vi "Test Comm Multi.vi"() -> ()   [LabVIEW 2021]
uses:
  ChannelCommon/typedef/FIFO Config.ctl
  ChannelCommon/ChannelCommon.lvlib
  CIFChannels/Typedef/Direction.ctl
  CIFChannels/CIFChannels.lvclass
  ChannelCommon/typedef/TimeStamps.ctl
  CIF_Fifo_U8_Multi.lvclass
  ChannelCommon/typedef/New FIFO Instance Configuration.ctl
  FIFO_U8/CIF_NIChn_Fifo_U8.lvclass
  D:/dev/Packages/CIF_Channels_Core/src/CIF_NIChn/FIFO_U8/CIF_NIChn_Fifo_U8.lvclass
  D:/dev/Packages/CIF_Channels_Core/src/CIF_NIChn/NIChn/CIF_NIChn.lvclass
  D:/dev/Packages/CIF_Channels_Core/src/CIFChannels/CIFChannels.lvclass
  D:/dev/Packages/CIF_Channels_Core/src/CIF_NIChn/FIFO_U8_Multi/CIF_Fifo_U8_Multi.lvclass
panel:
  out "status":string
  out "pass":bool
  out "error out":errorcluster
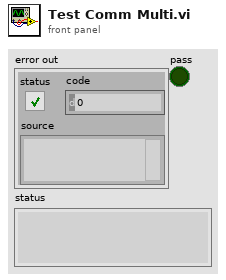
[diagram p1: front panel]
types:
  T1 = typedef "CIFChannels.lvclass/Direction.ctl" = enum16{"Publisher", "Subscriber"}
  T2 = typedef "ChannelCommon.lvlib/New FIFO Instance Configuration.ctl" = cluster{"Primary":bool, "Backpressure":bool, "Message/FIFO Override":u32}
  T3 = typedef "ChannelCommon.lvlib/TimeStamps.ctl" = cluster{"ClockID":u8, "T0":i64, "T_Out":i64}
  T4 = typedef "ChannelCommon.lvlib/FIFO Config.ctl" = cluster{"Max Bytes/Msg":u64, "Max Msg/FIFO":u64, "Flags":u64}
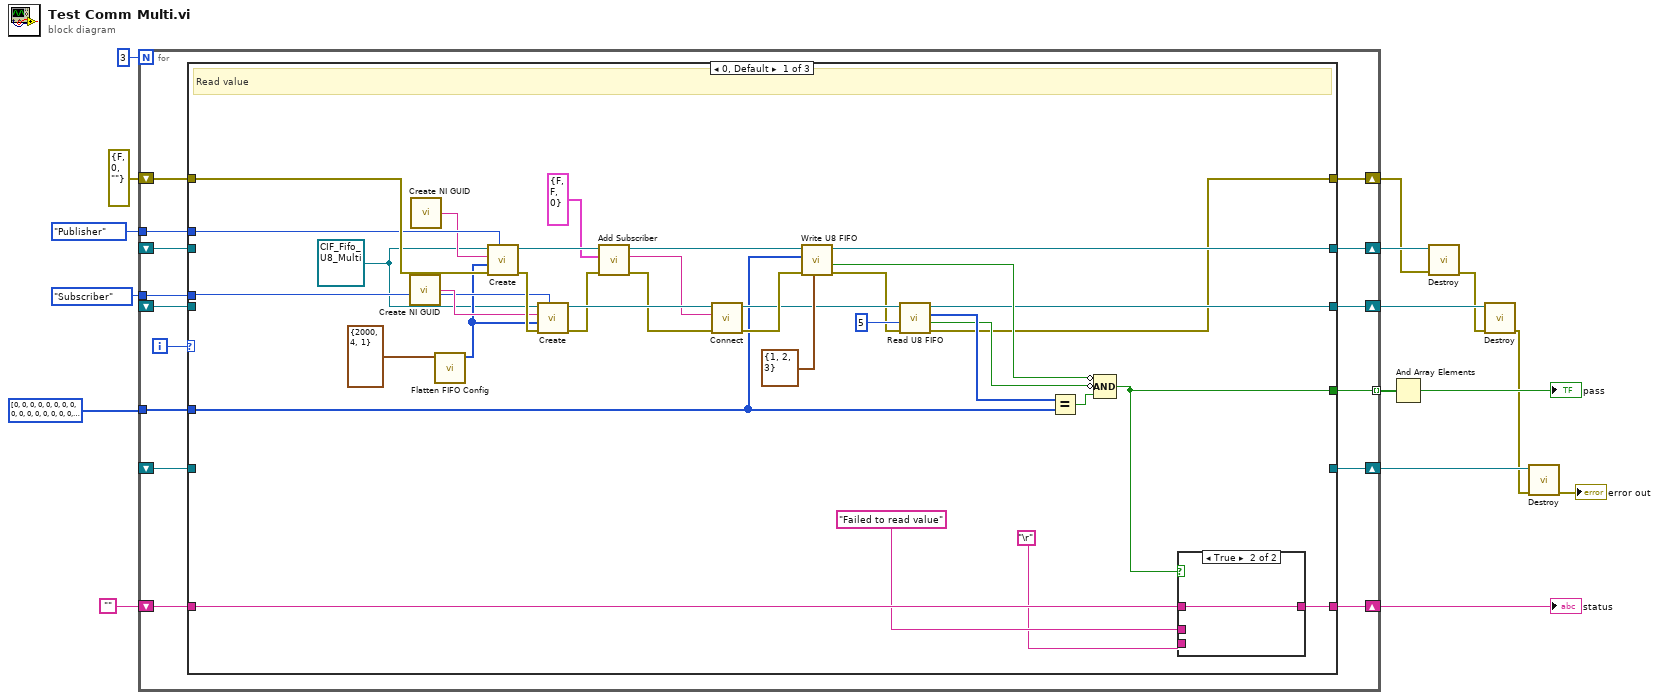
[diagram p0: block diagram]
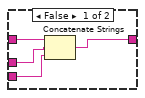
[diagram p2: hidden frame]
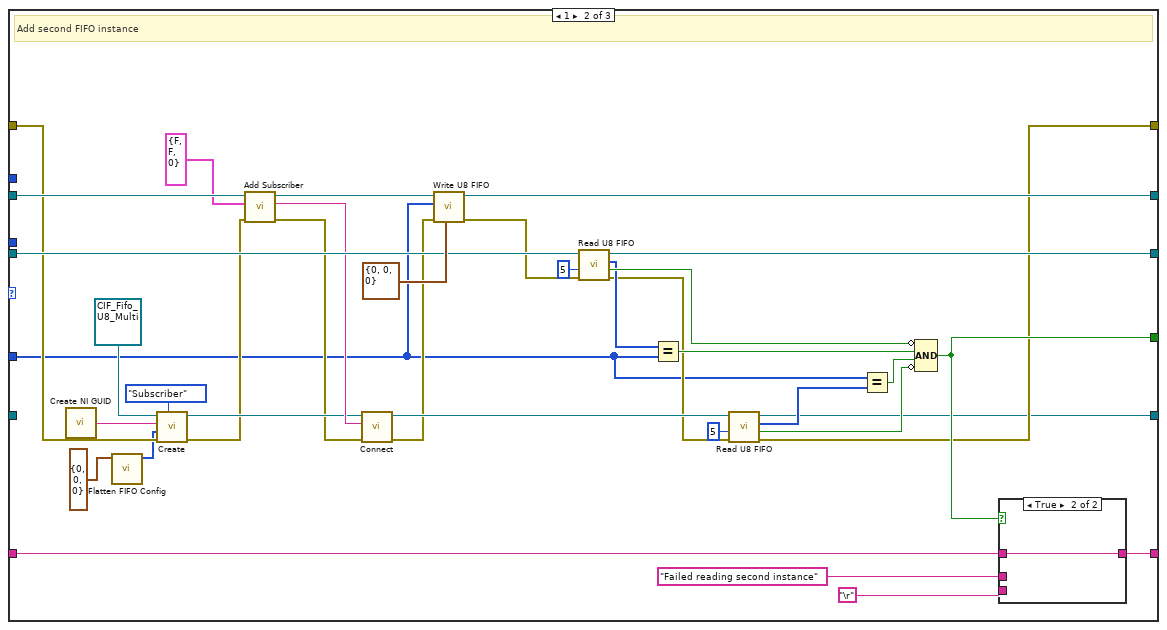
[diagram p3: hidden frame]
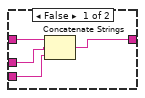
[diagram p4: hidden frame]
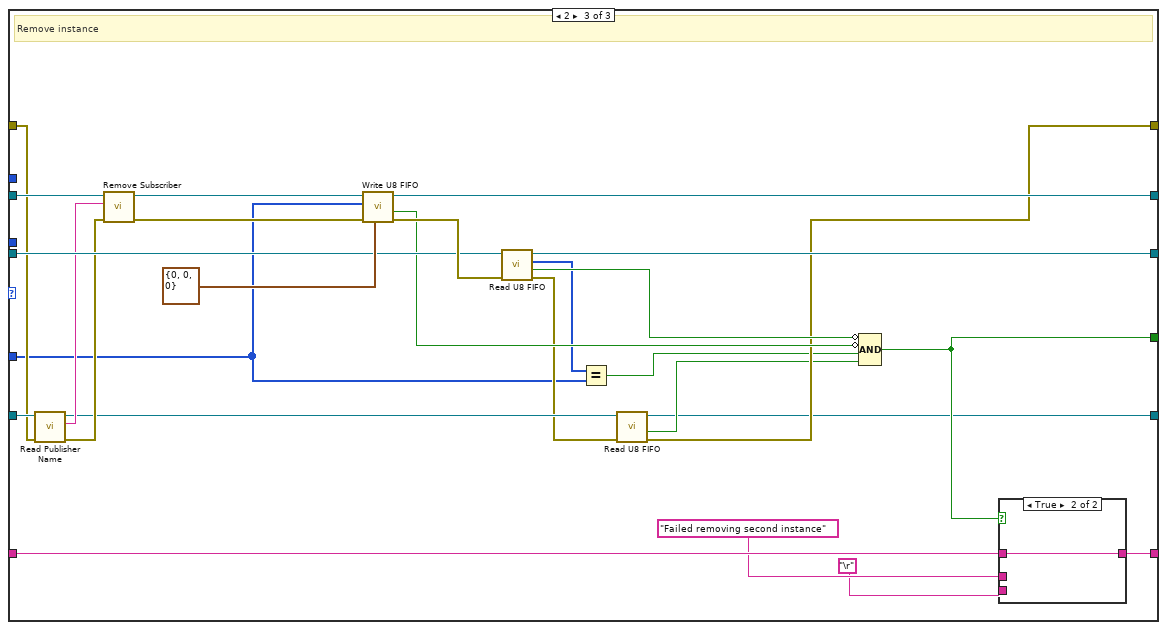
[diagram p5: hidden frame]
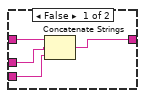
[diagram p6: hidden frame]
diagram:
  n1 = for {
    N: 3 -> [_]
    tunnel: [w31] -> w16 mode=indexing
    shift-right: [w22] -> w6
    shift-left: errorcluster {"status"=FALSE, "code"=0, "source"=""} ("error out") -> [w30]
    shift-right: [w27] -> w12
    shift-left: "" -> [w28]
    tunnel: Direction."Subscriber" ("Direction") -> [w26]
    tunnel: Direction."Publisher" ("Direction") -> [w25]
    shift-right: [w24] -> w8
    shift-left: _ -> [w20]
    shift-right: [w23] -> w7
    shift-left: _ -> [w21]
    tunnel: u8[] [0, 0, 0, 0, 0, 0, 0, 0, 0, 0, 0, 0, 0, 0, 0, 0, 0, 0, 0, 0, 0, 0, 0, 0, 0, 0, 0, 0, 0, 0, 0, 0, 0, 0, 0, 0, 0, 0, 0, 0, 0, 0, 0, 0, 0, 0, 0, 0, 0, 0, 0, 0, 0, 0, 0, 0, 0, 0, 0, 0, 0, 0, 0, 0, 0, 0, 0, 0, 0, 0, 0, 0, 0, 0, 0, 0, 0, 0, 0, 0, 0, 0, 0, 0, 0, 0, 0, 0, 0, 0, 0, 0, 0, 0, 0, 0, 0, 0, 0, 0, 0, 0, 0, 0, 0, 0, 0, 0, 0, 0, 0, 0, 0, 0, 0, 0, 0, 0, 0, 0, 0, 0, 0, 0, 0, 0, 0, 0, 0, 0, 0, 0, 0, 0, 0, 0, 0, 0, 0, 0, 0, 0, 0, 0, 0, 0, 0, 0, 0, 0, 0, 0, 0, 0, 0, 0, 0, 0, 0, 0, 0, 0, 0, 0, 0, 0, 0, 0, 0, 0, 0, 0, 0, 0, 0, 0, 0, 0, 0, 0, 0, 0, 0, 0, 0, 0, 0, 0, 0, 0, 0, 0, 0, 0, 0, 0, 0, 0, 0, 0, 0, 0, 0, 0, 0, 0, 0, 0, 0, 0, 0, 0, 0, 0, 0, 0, 0, 0, 0, 0, 0, 0, 0, 0, 0, 0, 0, 0, 0, 0, 0, 0, 0, 0, 0, 0, 0, 0, 0, 0, 0, 0, 0, 0, 0, 0, 0, 0, 0, 0, 0, 0, 0, 0, 0, 0, 0, 0, 0, 0, 0, 0, 0, 0, 0, 0, 0, 0, 0, 0, 0, 0, 0, 0, 0, 0, 0, 0, 0, 0, 0, 0, 0, 0, 0, 0, 0, 0, 0, 0, 0, 0, 0, 0, 0, 0, 0, 0, 0, 0, 0, 0, 0, 0, 0, 0, 0, 0, 0, 0, 0, 0, 0, 0, 0, 0, 0, 0, 0, 0, 0, 0, 0, 0, 0, 0, 0, 0, 0, 0, 0, 0, 0, 0, 0, 0, 0, 0, 0, 0, 0, 0, 0, 0, 0, 0, 0, 0, 0, 0, 0, 0, 0, 0, 0, 0, 0, 0, 0, 0, 0, 0, 0, 0, 0, 0, 0, 0, 0, 0, 0, 0, 0, 0, 0, 0, 0, 0, 0, 0, 0, 0, 0, 0, 0, 0, 0, 0, 0, 0, 0, 0, 0, 0, 0, 0, 0, 0, 0, 0, 0, 0, 0, 0, 0, 0, 0, 0, 0, 0, 0, 0, 0, 0, 0, 0, 0, 0, 0, 0, 0, 0, 0, 0, 0, 0, 0, 0, 0, 0, 0, 0, 0, 0, 0, 0, 0, 0, 0, 0, 0, 0, 0, 0, 0, 0, 0, 0, 0, 0, 0, 0, 0, 0, 0, 0, 0, 0, 0, 0, 0, 0, 0, 0, 0, 0, 0, 0, 0, 0, 0, 0, 0, 0, 0, 0, 0, 0, 0, 0, 0, 0, 0, 0, 0, 0, 0, 0, 0, 0, 0, 0, 0, 0, 0, 0, 0, 0, 0, 0, 0, 0, 0, 0, 0, 0, 0, 0, 0, 0, 0, 0, 0, 0, 0, 0, 0, 0, 0, 0, 0, 0, 0, 0, 0, 0, 0, 0, 0, 0, 0, 0, 0, 0, 0, 0, 0, 0, 0, 0, 0, 0, 0, 0, 0, 0, 0, 0, 0, 0, 0, 0, 0, 0, 0, 0, 0, 0, 0, 0, 0, 0, 0, 0, 0, 0, 0, 0, 0, 0, 0, 0, 0, 0, 0, 0, 0, 0, 0, 0, 0, 0, 0, 0, 0, 0, 0, 0, 0, 0, 0, 0, 0, 0, 0, 0, 0, 0, 0, 0, 0, 0, 0, 0, 0, 0, 0, 0, 0, 0, 0, 0, 0, 0, 0, 0, 0, 0, 0, 0, 0, 0, 0, 0, 0, 0, 0, 0, 0, 0, 0, 0, 0, 0, 0, 0, 0, 0, 0, 0, 0, 0, 0, 0, 0, 0, 0, 0, 0, 0, 0, 0, 0, 0, 0, 0, 0, 0, 0, 0, 0, 0, 0, 0, 0, 0, 0, 0, 0, 0, 0, 0, 0, 0, 0, 0, 0, 0, 0, 0, 0, 0, 0, 0, 0, 0, 0, 0, 0, 0, 0, 0, 0, 0, 0, 0, 0, 0, 0, 0, 0, 0, 0, 0, 0, 0, 0, 0, 0, 0, 0, 0, 0, 0, 0, 0, 0, 0, 0, 0, 0, 0, 0, 0, 0, 0, 0, 0, 0, 0, 0, 0, 0, 0, 0, 0, 0, 0, 0, 0, 0, 0, 0, 0, 0, 0, 0, 0, 0, 0, 0, 0, 0, 0, 0, 0, 0, 0, 0, 0, 0, 0, 0, 0, 0, 0, 0, 0, 0, 0, 0, 0, 0, 0, 0, 0, 0, 0, 0, 0, 0, 0, 0, 0, 0, 0, 0, 0, 0, 0, 0, 0, 0, 0, 0, 0, 0, 0, 0, 0, 0, 0, 0, 0, 0, 0, 0, 0, 0, 0, 0, 0, 0, 0, 0, 0, 0, 0, 0, 0, 0, 0, 0, 0, 0, 0, 0, 0, 0, 0, 0, 0, 0, 0, 0, 0, 0, 0, 0, 0, 0, 0, 0, 0, 0, 0, 0, 0, 0, 0, 0, 0, 0, 0, 0, 0, 0, 0, 0, 0, 0, 0, 0, 0, 0, 0, 0, 0, 0, 0, 0, 0, 0, 0, 0, 0, 0, 0, 0, 0, 0, 0, 0, 0, 0, 0, 0, 0, 0, 0, 0, 0, 0, 0, 0, 0, 0, 0, 0, 0, 0, 0, 0, 0, 0, 0, 0, 0, 0, 0, 0, 0, 0, 0, 0, 0, 0, 0, 0, 0, 0, 0, 0, 0, 0, 0, 0, 0, 0, 0, 0, 0, 0, 0, 0, 0, 0, 0, 0, 0, 0, 0, 0, 0, 0, 0, 0, 0, 0, 0, 0, 0, 0, 0, 0, 0, 0, 0, 0, 0, 0, 0, 0, 0, 0, 0, 0, 0, 0, 0, 0, 0, 0, 0, 0, 0, 0, 0, 0, 0, 0, 0, 0, 0, 0, 0, 0, 0, 0, 0, 0, 0, 0, 0, 0, 0, 0, 0, 0, 0, 1] ("Data in") -> [w19]
    shift-right: [w17] -> w4
    shift-left: _ -> [w18]
    i -> [w29]
    n2 = case shown="0, Default" w29 {
      tunnel: [w60 w103 w133] -> w31
      tunnel: w30 -> [w58 w86 w126]
      tunnel: [w41 w76 w118] -> w22
      tunnel: w28 -> [w65 w107 w139]
      tunnel: [w64 w106 w138] -> w27
      tunnel: w26 -> [w56 _ _]
      tunnel: w25 -> [w55 _ _]
      tunnel: [w43 w77 w130] -> w24
      tunnel: [w48 w95 w121] -> w23
      tunnel: w21 -> [_ w94 w129]
      tunnel: w20 -> [_ w96 w131]
      tunnel: w19 -> [w33 w75 w114]
      tunnel: w18 -> [_ _ w127]
      tunnel: [_ w71 w113] -> w17
      frame 0, Default {
        w40 = refnum<class "CIF_Fifo_U8_Multi.lvclass"> refnum ("CIF_DAQ_DVR_Multi.lvclass")
        # "Read value"
        n3 = call <vilib>:"Create NI GUID.vi"() -> ("NI GUID"=w57:string)
        n4 = call <vilib>:"Create NI GUID.vi"() -> ("NI GUID"=w53:string)
        n5 = call "Flatten FIFO Config.vi"("FIFO Config in"=T4 {"Max Bytes/Msg"=2000, "Max Msg/FIFO"=4, "Flags"=1}) -> ("Flattened FIFO Config"=w51:u8[])  [unwired: 10 in]
        n6 = call-dynamic "Create.vi"("Direction"=w55, "error in (no error)"=w58, "Custom Config Data"=w51, "Name"=w53, "CIF_Fifo_U8 in"=w40) -> ("error out"=w59:errorcluster, "CIF_Fifo_U8 out"=w39:refnum<class "CIF_Fifo_U8_Multi.lvclass">)  [unwired: 5 in]
        n7 = call-dynamic "Create.vi"("Direction"=w56, "error in (no error)"=w59, "Custom Config Data"=w51, "Name"=w57, "CIF_Fifo_U8 in"=w40) -> ("error out"=w36:errorcluster, "CIF_Fifo_U8 out"=w52:refnum<class "CIF_Fifo_U8_Multi.lvclass">)  [unwired: 5 in]
        n8 = call-dynamic "Add Subscriber.vi"("error in (no error)"=w36, "New FIFO Instance Config"=T2 {"Primary"=FALSE, "Backpressure"=FALSE, "Message/FIFO Override"=0}, "CIF_Fifo_U8 in"=w39) -> ("error out"=w35:errorcluster, "New Publisher"=w37:string, "CIF_Fifo_U8 out"=w38:refnum<class "CIF_Fifo_U8_Multi.lvclass">)  [unwired: 6 in]
        n9 = call-dynamic "Connect.vi"("error in (no error)"=w35, "Connection Name"=w37, "CIFTag in"=w52) -> ("error out"=w50:errorcluster, "CIFTag out"=w46:refnum<class "CIF_Fifo_U8_Multi.lvclass">)  [unwired: 7 in]
        n10 = call-dynamic "Write U8 FIFO.vi"("FIFO Timestamps"=T3 {"ClockID"=1, "T0"=2, "T_Out"=3}, "error in (no error)"=w50, "Data in"=w33, "CIF_Fifo_U8 in"=w38) -> ("error out"=w32:errorcluster, "timed out?"=w47:bool, "CIF_Fifo_U8 out"=w48:refnum<class "CIF_Fifo_U8_Multi.lvclass">)  [unwired: 4 in, 1 out]
        n11 = call-dynamic "Read U8 FIFO.vi"("error in (no error)"=w32, "Timeout (ms)"=5, "CIFFIFO in"=w46) -> ("error out"=w41:errorcluster, "timed out?"=w42:bool, "Data out"=w44:u8[], "CIFFIFO out"=w43:refnum<class "CIF_Fifo_U8_Multi.lvclass">)  [unwired: 4 in, 1 out]
        n12 = Equal?(x=w44, y=w33) -> (x = y?=w61:bool)
        n13 = Compound Arithmetic op=AND(invert w47, invert w42, w61) -> (w60:bool)
        n14 = case shown="True" w60 {
          tunnel: w65 -> [w69 w70]
          tunnel: [w66 w70] -> w64
          tunnel: "Failed to read value" -> [w68 _]
          tunnel: "\r" -> [w67 _]
          frame False {
            n15 = Concatenate Strings(w69, w68, w67) -> (w66:string)
          }
          frame True {
          }
        }
      }
      frame 1 {
        # "Add second FIFO instance"
        n16 = call <vilib>:"Create NI GUID.vi"() -> ("NI GUID"=w91:string)
        n17 = call "Flatten FIFO Config.vi"("FIFO Config in"=T4 {"Max Bytes/Msg"=0, "Max Msg/FIFO"=0, "Flags"=0}) -> ("Flattened FIFO Config"=w85:u8[])  [unwired: 10 in]
        n18 = call-dynamic "Create.vi"("Direction"=Direction."Subscriber", "error in (no error)"=w86, "Custom Config Data"=w85, "Name"=w91, "CIF_Fifo_U8 in"=refnum<class "CIF_Fifo_U8_Multi.lvclass"> refnum ("CIF_DAQ_DVR_Multi.lvclass")) -> ("error out"=w87:errorcluster, "CIF_Fifo_U8 out"=w89:refnum<class "CIF_Fifo_U8_Multi.lvclass">)  [unwired: 5 in]
        n19 = call-dynamic "Add Subscriber.vi"("error in (no error)"=w87, "New FIFO Instance Config"=T2 {"Primary"=FALSE, "Backpressure"=FALSE, "Message/FIFO Override"=0}, "CIF_Fifo_U8 in"=w94) -> ("error out"=w88:errorcluster, "New Publisher"=w90:string, "CIF_Fifo_U8 out"=w93:refnum<class "CIF_Fifo_U8_Multi.lvclass">)  [unwired: 6 in]
        n20 = call-dynamic "Connect.vi"("error in (no error)"=w88, "Connection Name"=w90, "CIFTag in"=w89) -> ("error out"=w80:errorcluster, "CIFTag out"=w81:refnum<class "CIF_Fifo_U8_Multi.lvclass">)  [unwired: 7 in]
        n21 = call-dynamic "Write U8 FIFO.vi"("FIFO Timestamps"=T3 {"ClockID"=0, "T0"=0, "T_Out"=0}, "error in (no error)"=w80, "Data in"=w75, "CIF_Fifo_U8 in"=w93) -> ("error out"=w74:errorcluster, "CIF_Fifo_U8 out"=w95:refnum<class "CIF_Fifo_U8_Multi.lvclass">)  [unwired: 4 in, 2 out]
        n22 = call-dynamic "Read U8 FIFO.vi"("error in (no error)"=w74, "Timeout (ms)"=5, "CIFFIFO in"=w96) -> ("error out"=w78:errorcluster, "timed out?"=w99:bool, "Data out"=w98:u8[], "CIFFIFO out"=w77:refnum<class "CIF_NIChn_Fifo_U8.lvclass">)  [unwired: 4 in, 1 out]
        n23 = Equal?(x=w98, y=w75) -> (x = y?=w101:bool)
        n24 = call-dynamic "Read U8 FIFO.vi"("error in (no error)"=w78, "Timeout (ms)"=5, "CIFFIFO in"=w81) -> ("error out"=w76:errorcluster, "timed out?"=w72:bool, "Data out"=w79:u8[], "CIFFIFO out"=w71:refnum<class "CIF_Fifo_U8_Multi.lvclass">)  [unwired: 4 in, 1 out]
        n25 = Equal?(x=w75, y=w79) -> (x = y?=w102:bool)
        n26 = Compound Arithmetic op=AND(invert w99, w101, w102, invert w72) -> (w103:bool)
        n27 = case shown="True" w103 {
          tunnel: w107 -> [w111 w112]
          tunnel: [w108 w112] -> w106
          tunnel: "Failed reading second instance" -> [w110 _]
          tunnel: "\r" -> [w109 _]
          frame False {
            n28 = Concatenate Strings(w111, w110, w109) -> (w108:string)
          }
          frame True {
          }
        }
      }
      frame 2 {
        # "Remove instance"
        n29 = call "Read Publisher Name.vi"("error in (no error)"=w126, "CIFChannels in"=w127) -> ("error out"=w123:errorcluster, "Publisher Name"=w125:string, "CIFChannels out"=w120:refnum<class "CIF_Fifo_U8_Multi.lvclass">)  [unwired: 7 in]
        n30 = call-dynamic "Remove Subscriber.vi"("error in (no error)"=w123, "Publisher to Remove"=w125, "CIF_Fifo_U8 in"=w129) -> ("error out"=w124:errorcluster, "CIF_Fifo_U8 out"=w128:refnum<class "CIF_Fifo_U8_Multi.lvclass">)  [unwired: 7 in]
        n31 = call-dynamic "Write U8 FIFO.vi"("FIFO Timestamps"=T3 {"ClockID"=0, "T0"=0, "T_Out"=0}, "error in (no error)"=w124, "Data in"=w114, "CIF_Fifo_U8 in"=w128) -> ("error out"=w135:errorcluster, "timed out?"=w122:bool, "CIF_Fifo_U8 out"=w121:refnum<class "CIF_Fifo_U8_Multi.lvclass">)  [unwired: 4 in, 1 out]
        n32 = call-dynamic "Read U8 FIFO.vi"("error in (no error)"=w135, "CIFFIFO in"=w131) -> ("error out"=w119:errorcluster, "timed out?"=w134:bool, "Data out"=w117:u8[], "CIFFIFO out"=w130:refnum<class "CIF_NIChn_Fifo_U8.lvclass">)  [unwired: 5 in, 1 out]
        n33 = Equal?(x=w117, y=w114) -> (x = y?=w116:bool)
        n34 = call-dynamic "Read U8 FIFO.vi"("error in (no error)"=w119, "CIFFIFO in"=w120) -> ("error out"=w118:errorcluster, "timed out?"=w115:bool, "CIFFIFO out"=w113:refnum<class "CIF_Fifo_U8_Multi.lvclass">)  [unwired: 5 in, 2 out]
        n35 = Compound Arithmetic op=AND(invert w134, invert w122, w116, w115) -> (w133:bool)
        n36 = case shown="True" w133 {
          tunnel: w139 -> [w143 w144]
          tunnel: [w140 w144] -> w138
          tunnel: "Failed removing second instance" -> [w142 _]
          tunnel: "\r" -> [w141 _]
          frame False {
            n37 = Concatenate Strings(w143, w142, w141) -> (w140:string)
          }
          frame True {
          }
        }
      }
    }
  }
  "status" <- w12
  n38 = And Array Elements(Boolean array=w16) -> (logical AND=→"pass":bool)
  n39 = call-dynamic "Destroy.vi"("error in (no error)"=w6, "CIF_Fifo_U8 in"=w7) -> ("error out"=w5:errorcluster)  [unwired: 8 in, 1 out]
  n40 = call-dynamic "Destroy.vi"("error in (no error)"=w5, "CIFFIFO in"=w8) -> ("error out"=w3:errorcluster)  [unwired: 8 in, 1 out]
  n41 = call-dynamic "Destroy.vi"("error in (no error)"=w3, "CIF_Fifo_U8 in"=w4) -> ("error out"=→"error out":errorcluster)  [unwired: 8 in, 1 out]
